vi "Read DIO Mode.vi"(8 "error in":errorcluster, 11 "mode in":refnum<class "Mode.lvclass">) -> (0 "error out":errorcluster, 2 "DIO mode":u32, 3 "mode out":refnum<class "Mode.lvclass">)   [LabVIEW 2017, in "Scan Engine Scripting.lvlib" / "Mode.lvclass"]
uses:
  Mode.lvclass
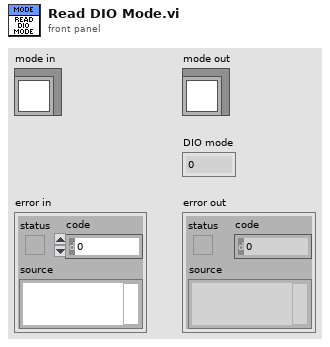
[diagram p1: front panel]
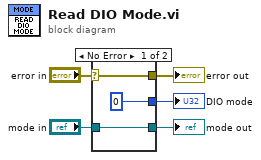
[diagram p0: block diagram]
diagram:
  n1 = case shown="No Error" "error in" {
    selector: "error in" -> [w7 w10]
    tunnel: [w7 w10] -> w4
    tunnel: [w8 w9] -> w2
    tunnel: "mode in" -> [w8 w9]
    tunnel: [u32 0 ("DIO mode") _] -> w1
    frame No Error {
    }
    frame Error {
    }
  }
  "error out" <- w4
  "mode out" <- w2
  "DIO mode" <- w1
